vi "Untitled 2.vi"() -> ()   [LabVIEW 2019]
panel:
  out "Boolean 3":bool
  out "Boolean":bool
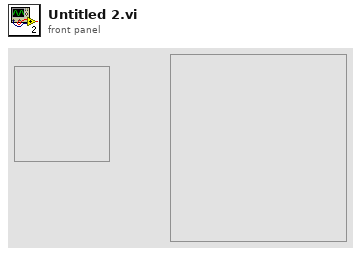
[diagram p1: front panel]
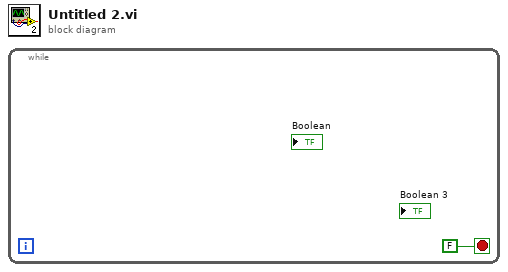
[diagram p0: block diagram]
diagram:
  n1 = while {
    stop <- FALSE stop-if-true
  }
